vi "Read P.vi"(8 "error in (no error)":errorcluster, 11 "CRDS Data in":refnum<class "CRDS Data.lvclass">) -> (0 "error out":errorcluster, 2 "P":sgl[](array[numeric]), 3 "CRDS Data out":refnum<class "CRDS Data.lvclass">)   [LabVIEW 2011]
doc: "Retrieve the pressures stored in the CRDS Data class."
uses:
  CRDS Data.lvclass
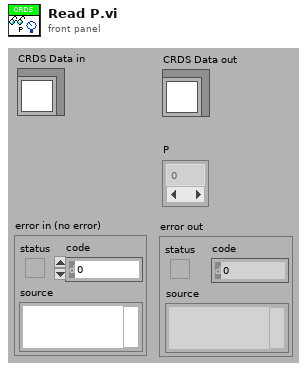
[diagram p1: front panel]
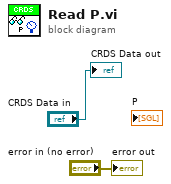
[diagram p0: block diagram]
diagram:
  "error out" <- "error in (no error)"
  "CRDS Data out" <- "CRDS Data in"
